vi "drive robot.vi"() -> ()   [LabVIEW 2018]
panel:
  in  "Max Allowed Speed [0, 1] (0)":dbl
  out "error out":errorcluster
  in  "stop":bool
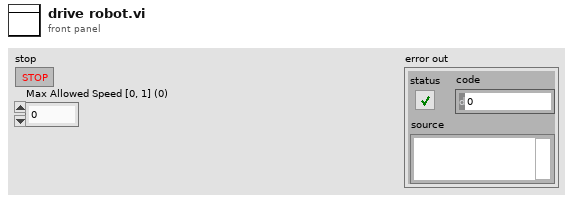
[diagram p1: front panel]
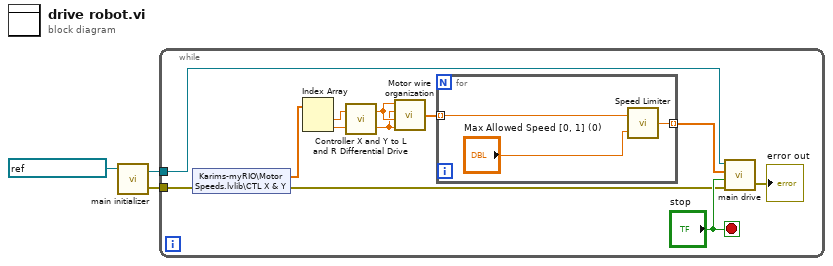
[diagram p0: block diagram]
diagram:
  n1 = call "main initializer.vi"("VISA resource name in"=refnum<visa-resource-name> "ASRL1::INSTR") -> ("error out"=w1:errorcluster, "VISA resource name out"=w2:refnum<visa-resource-name>)  [unwired: 2 in]
  n2 = while {
    tunnel: w2 -> [w15]
    tunnel: w1 -> [w13]
    stop <- "stop" stop-if-true
    n3 = shared-variable "Karims-myRIO\\Motor Speeds.lvlib\\CTL X & Y"(error in=w13) -> (w9:dbl[], error out=w12:errorcluster)
    n4 = Index Array(array=w9) -> (element #1=w8:dbl, element #2=w7:dbl)  [unwired: 2 in]
    n5 = call "Controller X and Y to L and R Differential Drive.vi"("Controller Y-Axis"=w7, "Controller X-Axis"=w8) -> ("Right Side Motors"=w4:dbl, "Left Side Motors"=w5:dbl)
    n6 = call "Motor wire organization.vi"("Motor Speed 1 (Right Rear)"=w4, "Motor Speed 2 (Left Rear)"=w5, "Motor Speed 3 (Right Front)"=w4, "Motor Speed 4 (Left Front)"=w5) -> ("Array of Motor Speeds"=w6:dbl[])  [unwired: 6 in]
    n7 = for {
      tunnel: w6 -> [w17] mode=indexing
      tunnel: [w18] -> w10 mode=indexing
      n8 = call "Speed Limiter.vi"("Max Allowed Speed [0, 1] (0)"="Max Allowed Speed [0, 1] (0)", "Raw Speed In"=w17) -> ("Speed Limited Output"=w18:dbl)
    }
    n9 = call "main drive.vi"("error in (no error)"=w12, "Stop? (Speeds = 0?)"="stop", "Array of Motor Speeds"=w10, "VISA resource name"=w15) -> ("error out"=→"error out":errorcluster)  [unwired: 1 out]
  }
